vi "DIMAQ ReadFile.vi"   [LabVIEW 2014]
panel:
  # "Snippet for dropping: ReadFile with IMAQ Create"
types:
  T1 = typedef "IMAQ Image.ctl" = refnum<image>
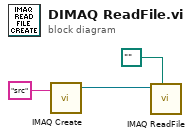
[diagram p0: block diagram]
diagram:
  n1 = call "IMAQ Create"("Image Name"="src") -> ("New Image"=w2:T1)  [unwired: 4 in, 1 out]
  n2 = call "IMAQ ReadFile"("File Path"=path "", "Image"=w2) -> ()  [unwired: 5 in, 5 out]
